vi "SwitchedACIR.vi"(4 "ACIR ClassName":string="Hioki BT4560B.lvclass", 5 "Setting":T1={"Freq"=1000.0, "Range"=enum."10m Ohm", "Measurements"=enum."Impedence"} {"Freq" min=0.1 max=1050.0 step=0.01 format="%_5e"}, 6 "ACIR Ref":string, 7 "Connection(s)":string, 8 "error in":errorcluster, 9 "Switch Ref":string, 10 "Switch ClassName":string="Hioki9002.lvclass", 11 "Base Path":path=path "C:/GitHub/OOP_OPC UA/Sequence/CodeModules/HAL/Concrete") -> (0 "error out":errorcluster={"status"=TRUE, "code"=-1073807346, "source"="VISA Open in APS-7000 Series.lvlib:Initialize.vi->Concrete.lvlib:APS7050.lvclass:Initialise.vi->Check objects.vi"}, 3 "Measurements":dbl)   [LabVIEW 2021]
uses:
  HAL/Harware Abstraction/Switch/Switch.lvclass
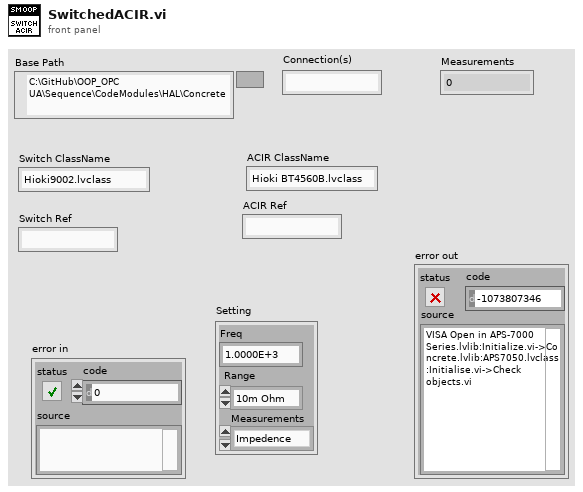
[diagram p1: front panel]
types:
  T1 = cluster{"Freq":dbl, "Range":enum16{"3m Ohm", "10m Ohm", "100m Ohm"}, "Measurements":enum16{"Impedence", "Phase Angle", "OCV"}}
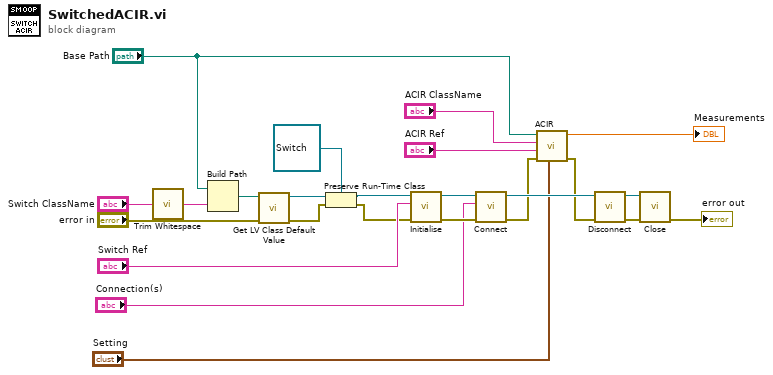
[diagram p0: block diagram]
diagram:
  n1 = call <vilib>:"Trim Whitespace.vi"("string"="Switch ClassName") -> ("trimmed string"=w22:string)  [unwired: 1 in]
  n2 = Build Path(base path="Base Path", name or relative path=w22) -> (appended path=w20:path)
  n3 = call <vilib>:"Get LV Class Default Value.vi"("error in (no error)"="error in", "class path"=w20) -> ("error out"=w19:errorcluster, "object"=w23:refnum<class>)  [unwired: 8 in]
  n4 = Preserve Run-Time Class(object in=w23, error in=w19, 2:refnum<class "Switch.lvclass"> refnum ("HAL.lvlib:Switch.lvclass")) -> (object out=w17:refnum<class "Switch.lvclass">, error out=w16:errorcluster)
  n5 = call-dynamic "Initialise.vi"("error in (no error)"=w16, "Instrument Ref"="Switch Ref", "Instrument in"=w17) -> ("error out"=w13:errorcluster, "Instrument out"=w12:refnum<class "Switch.lvclass">)  [unwired: 7 in]
  n6 = call-dynamic "Connect.vi"("error in (no error)"=w13, "Channel(s)"="Connection(s)", "Switch in"=w12) -> ("error out"=w7:errorcluster, "Switch out"=w8:refnum<class "Switch.lvclass">)  [unwired: 7 in]
  n7 = call "ACIR.vi"("Setting"="Setting", "error in"=w7, "ACIR Ref"="ACIR Ref", "ACIR ClassName"="ACIR ClassName", "Base Path"="Base Path") -> ("error out"=w6:errorcluster, "Measurements"=→"Measurements":dbl)  [unwired: 5 in]
  n8 = call-dynamic "Disconnect.vi"("error in (no error)"=w6, "Switch in"=w8) -> ("error out"=w11:errorcluster, "Switch out"=w10:refnum<class "Switch.lvclass">)  [unwired: 8 in]
  n9 = call-dynamic "Close.vi"("error in (no error)"=w11, "Instrument in"=w10) -> ("error out"=→"error out":errorcluster)  [unwired: 8 in, 1 out]
